vi "Handle Output.vi"(8 "error in":errorcluster, 11 "Plugin_Controller in":refnum<class "Plugin_Controller.lvclass">) -> (0 "error out":errorcluster, 3 "Plugin_Controller out":refnum<class "Plugin_Controller.lvclass">)   [LabVIEW 2020, in "Plugin.lvlib" / "Plugin_Controller.lvclass"]
doc: "Configures the output voltage, as it is changed from Sequencer."
uses:
  Plugin_Controller.lvclass
  C:/SVN_LabSys/labsys_lvcode/LabSys_SourceCode/builds/Libraries/LabSys Framework.lvlibp/Configurable Data Node/Configurable Data Node/Configurable Data Node.lvclass
  C:/SVN_LabSys/labsys_lvcode/LabSys_SourceCode/builds/Libraries/LabSys Framework.lvlibp/Data Node/Data Node/Data Node.lvclass
  builds/Libraries/Value Object Library.lvlibp/Double/Double.lvclass
  Drivers/Instrument Driver/Typedefs/Output Settings.ctl
  Channels/Output Channels/Output Channels.lvclass
  C:/SVN_LabSys/labsys_lvcode/LabSys_SourceCode/Plugin Template/Source/Code/Channels/Plugin_Channels.lvclass
  builds/Libraries/LabSys Framework.lvlibp/Configurable Data Node/Configurable Data Node/Read Module Configuration.vi
  builds/Libraries/LabSys Framework.lvlibp/Data Node/Data Node/Read Data Subscriptions.vi
  builds/Libraries/LabSys Framework.lvlibp/Data Node/Data Node/Read Error Manager.vi
  builds/Libraries/LabSys Framework.lvlibp/Data Node/Data Node/Read Module Name.vi
  builds/Libraries/LabSys Framework.lvlibp/Data Distributor/Data Subscription/Read Variable Name.vi
  builds/Libraries/Value Object Library.lvlibp/Double/Read Value.vi
  Plugin_Driver/Plugin_Driver.lvclass
  builds/Libraries/LabSys Framework.lvlibp/Configuration Storage/Module Configuration/Module Configuration.lvclass
  builds/Libraries/LabSys Framework.lvlibp/Data Distributor/Data Subscription/Data Subscription.lvclass
  builds/Libraries/LabSys Framework.lvlibp/Error Manager/Error Manager/Error Manager.lvclass
  UI_Class/Plugin_UI.lvclass
  Drivers/Instrument Driver/Instrument Driver.lvclass
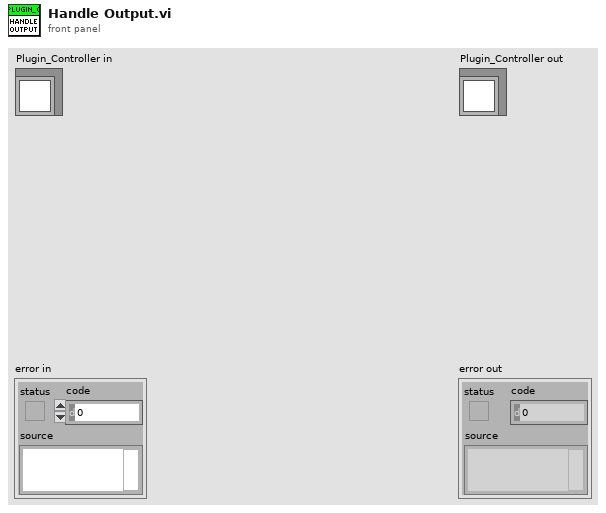
[diagram p1: front panel]
types:
  T1 = typedef "Plugin Instrument Driver.lvlib/Instrument Driver.lvclass/Output Settings.ctl" = cluster{"Voltage (V)":dbl}
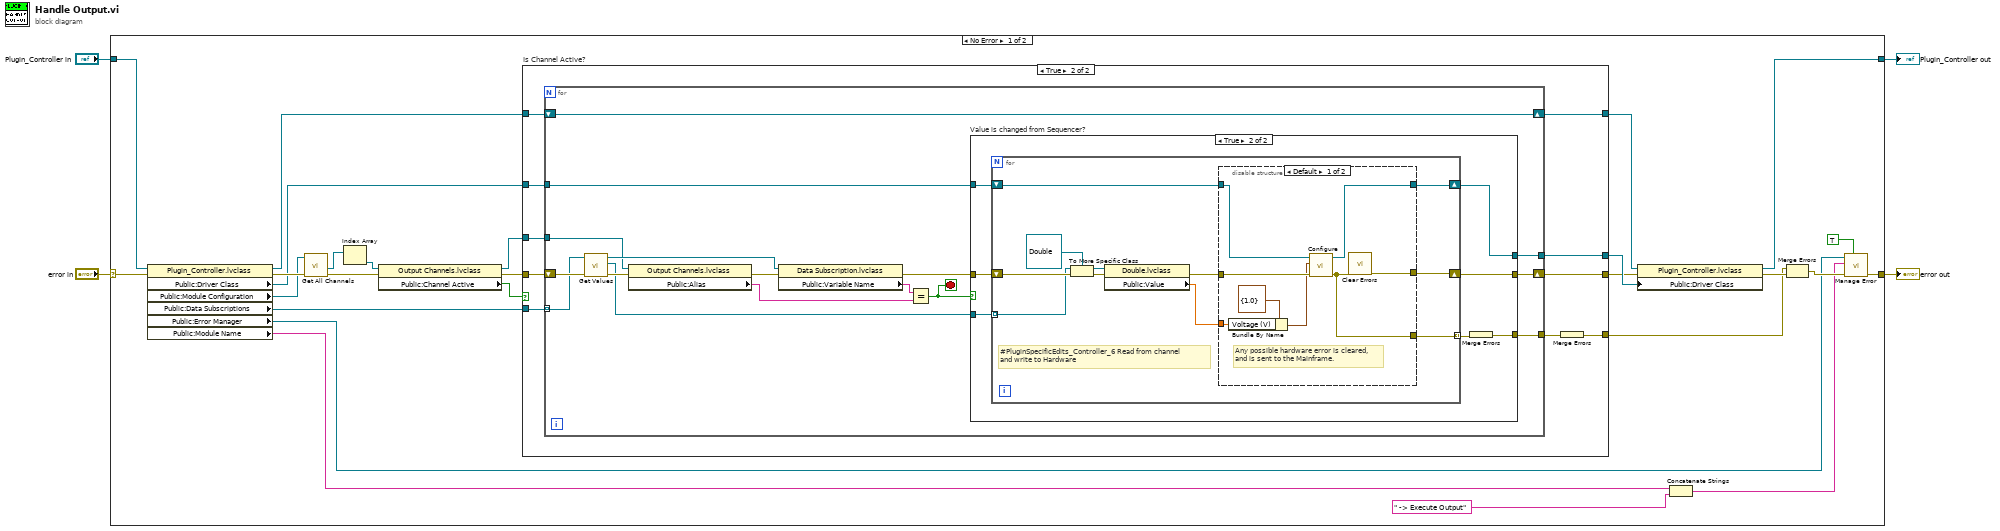
[diagram p0: block diagram]
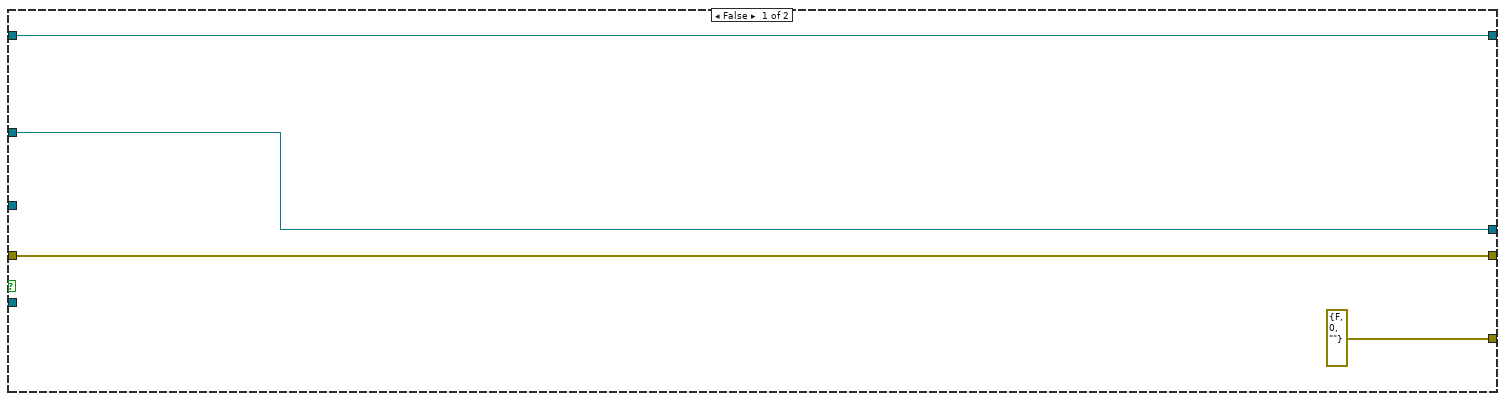
[diagram p2: hidden frame]
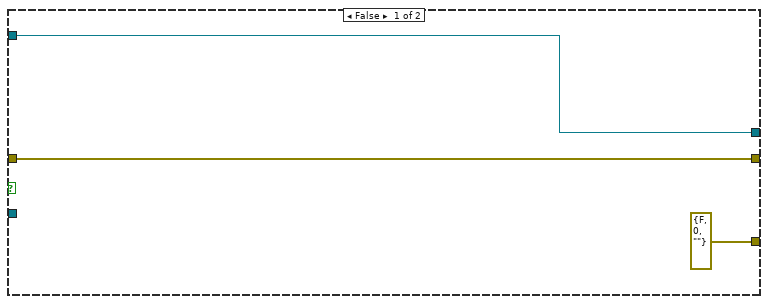
[diagram p3: hidden frame]
diagram:
  n1 = case shown="No Error" "error in" {
    selector: "error in" -> [w6 w93]
    tunnel: [w5 w93] -> w3
    tunnel: [w11 w92] -> w1
    tunnel: "Plugin_Controller in" -> [w12 w92]
    frame No Error {
      n2 = property class="Plugin_Controller.lvclass"(reference=w12, error in=w6) -> (reference out=w23:refnum<class "Plugin_Controller.lvclass">, error out=w30:errorcluster, "Public:Driver Class"=w24:refnum<class "Plugin_Driver.lvclass">, "Public:Module Configuration"=w29:refnum<class "Module Configuration.lvclass">, "Public:Data Subscriptions"=w20:refnum<class "Data Subscription.lvclass">[], "Public:Error Manager"=w8:refnum<data-value>, "Public:Module Name"=w7:string)
      n3 = call "Get All Channels.vi"("error in (no error)"=w30, "Module Configuration"=w29) -> ("error out"=w26:errorcluster, "Output Channels[]"=w27:refnum<class "Output Channels.lvclass">[])  [unwired: 5 in, 3 out]
      n4 = Index Array(array=w27) -> (element=w28:refnum<class "Output Channels.lvclass">)  [unwired: 1 in]
      n5 = property class="Output Channels.lvclass"(reference=w28, error in=w26) -> (reference out=w21:refnum<class "Output Channels.lvclass">, error out=w22:errorcluster, "Public:Channel Active"=w25:bool)
      n6 = case "Is Channel Active?" shown="True" w25 {
        tunnel: w24 -> [w33 w44]
        tunnel: w23 -> [w34 w43]
        tunnel: w22 -> [w32 w42]
        tunnel: w21 -> [_ w41]
        tunnel: w20 -> [_ w40]
        tunnel: [w34 w39] -> w16
        tunnel: [w33 w38] -> w15
        tunnel: [w32 w37] -> w14
        tunnel: [errorcluster {"status"=FALSE, "code"=0, "source"=""} ("error IO") w35] -> w13
        frame False {
        }
        frame True {
          n7 = for {
            tunnel: w44 -> [w49]
            shift-right: [w47] -> w39
            shift-left: w43 -> [w47]
            shift-right: [w48] -> w37
            shift-left: w42 -> [w55]
            tunnel: w41 -> [w54]
            tunnel: w40 -> [w53] mode=indexing
            tunnel: [w46] -> w38
            tunnel: [w45] -> w36
            stop <- w51 stop-if-true
            n8 = call-dynamic "Get Values.vi"("error in (no error)"=w55, "Data Subscription in"=w53) -> ("error out"=w60:errorcluster, "Values"=w50:refnum<class "Value.lvclass">[], "Data Subscription out"=w57:refnum<class "Data Subscription.lvclass">)  [unwired: 7 in]
            n9 = property class="Output Channels.lvclass"(reference=w54, error in=w60) -> (error out=w59:errorcluster, "Public:Alias"=w56:string)  [unwired: 1 out]
            n10 = property class="Data Subscription.lvclass"(reference=w57, error in=w59) -> (error out=w52:errorcluster, "Public:Variable Name"=w58:string)  [unwired: 1 out]
            n11 = Equal?(x=w58, y=w56) -> (x = y?=w51:bool)
            n12 = case "Value is changed from Sequencer?" shown="True" w51 {
              tunnel: w52 -> [w62 w70]
              tunnel: w50 -> [_ w68]
              tunnel: w49 -> [w63 w69]
              tunnel: [w62 w66] -> w48
              tunnel: [w63 w65] -> w46
              tunnel: [errorcluster {"status"=FALSE, "code"=0, "source"=""} ("error IO") w64] -> w45
              frame False {
              }
              frame True {
                n13 = for {
                  shift-right: [w73] -> w66
                  shift-left: w70 -> [w78]
                  shift-right: [w74] -> w65
                  shift-left: w69 -> [w75]
                  tunnel: w68 -> [w77] mode=indexing
                  tunnel: [w72] -> w67 mode=indexing
                  # "#PluginSpecificEdits_Controller_6 Read from channel\nand write to Hardware"
                  n14 = To More Specific Class(target class=refnum<class "Double.lvclass"> refnum ("Value Object Library.lvlibp:Double.lvclass"), reference=w77, error in=w78) -> (specific class reference=w80:refnum<class "Double.lvclass">, error out=w79:errorcluster)
                  n15 = property class="Double.lvclass"(reference=w80, error in=w79) -> (error out=w76:errorcluster, "Public:Value"=w71:dbl)  [unwired: 1 out]
                  n16 = disable-structure shown="Default" {
                    disable-tunnel: w75 -> [w89 w91]
                    disable-tunnel: w76 -> [w88 w90]
                    disable-tunnel: [w87 w90] -> w73
                    disable-tunnel: [w86 w91] -> w74
                    disable-tunnel: [w85 w90] -> w72
                    disable-tunnel: w71 -> [w83 _]
                    frame condition #0 (active) {
                      # "Any possible hardware error is cleared,\nand is sent to the Mainframe."
                      n17 = Bundle By Name(cluster=T1 {"Voltage (V)"=1.0} ("Output Settings"), "Voltage (V)"=w83) -> (w82:T1)
                      n18 = call "Configure.vi"("error in"=w88, "Output Settings"=w82, "Plugin_Driver in"=w89) -> ("error out"=w85:errorcluster, "Plugin_Driver out"=w86:refnum<class "Plugin_Driver.lvclass">)  [unwired: 7 in]
                      n19 = call <vilib>:"Clear Errors.vi"("error in (no error)"=w85) -> ("error out"=w87:errorcluster)  [unwired: 5 in, 1 out]
                    }
                    frame condition #1 {
                    }
                  }
                }
                n20 = Merge Errors(w67) -> (w64:errorcluster)
              }
            }
          }
          n21 = Merge Errors(w36) -> (w35:errorcluster)
        }
      }
      n22 = property class="Plugin_Controller.lvclass"(reference=w16, error in=w14, "Public:Driver Class"=w15) -> (reference out=w11:refnum<class "Plugin_Controller.lvclass">, error out=w18:errorcluster)
      n23 = Concatenate Strings(w7, " -> Execute Output" ("Error Location")) -> (w9:string)
      n24 = Merge Errors(w13, w18) -> (w17:errorcluster)
      n25 = call "Manage Error.vi"("Clear Errors (F)"=TRUE, "error in (no error)"=w17, "Error Location"=w9, "Error Manager in"=w8) -> ("error out"=w5:errorcluster)  [unwired: 6 in, 1 out]
    }
    frame Error {
    }
  }
  "error out" <- w3
  "Plugin_Controller out" <- w1
